vi "20211224_00.vi"(1 "Side C":dbl caption="Side C(C邊)", 2 "Side B":dbl caption="Side B(B邊)", 3 "Side A":dbl caption="Side A(A邊)") -> (0 "Area":dbl caption="Area(面積)")   [LabVIEW 2019]
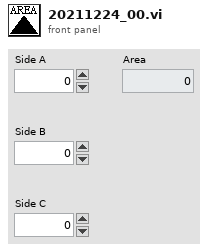
[diagram p1: front panel]
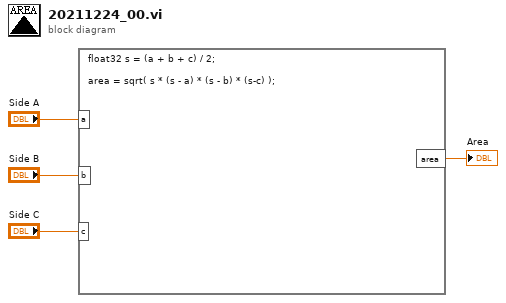
[diagram p0: block diagram]
diagram:
  n1 = formula code="float32 s = (a + b + c) / 2;\n\narea = sqrt( s * (s - a) * (s - b) * (s-c) );"("a"="Side A", "b"="Side B", "c"="Side C") -> ("area"=→"Area":dbl)
